vi "CAN task spawn.vi"(4 "error in (no error)":errorcluster, 7 "CANopen in":refnum<class "CANopen.lvclass">) -> (0 "error out":errorcluster, 3 "CANopen out":refnum<class "CANopen.lvclass">)   [LabVIEW 2024, in "canopen.lvlib" / "CANopen.lvclass"]
doc: "Spawns the \"CAN task\" VI with the provided arguments."
uses:
  CANopen.lvclass
  CANopen.lvclass/CANopen.ctl
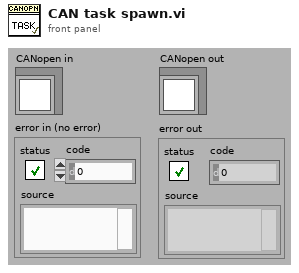
[diagram p1: front panel]
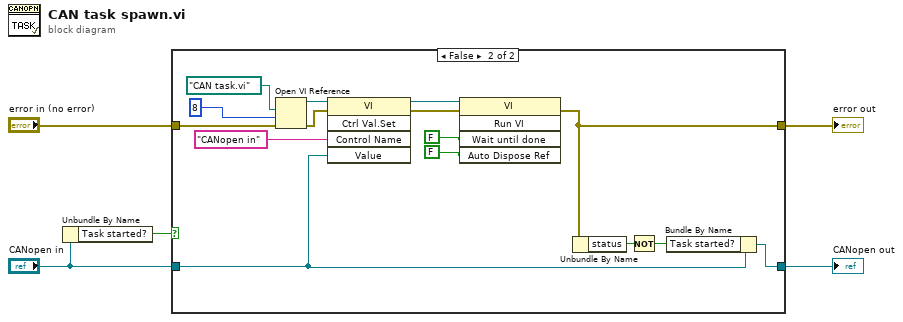
[diagram p0: block diagram]
diagram:
  n1 = Unbundle By Name("CANopen in") -> ("Task started?"=w1:bool)
  n2 = case shown="False" w1 {
    tunnel: "error in (no error)" -> [w7 w13]
    tunnel: "CANopen in" -> [w6 w12]
    tunnel: [w7 w11] -> w4
    tunnel: [w6 w8] -> w3
    frame True {
    }
    frame False {
      n3 = Open VI Reference(vi path=path "CAN task.vi", options=8, error in (no error)=w13) -> (vi reference=w18:refnum<vi>, error out=w19:errorcluster)  [unwired: 3 out]
      n4 = invoke class="VI" method="Ctrl Val.Set"(reference=w18, error in=w19, "Control Name"="CANopen in", "Value"=w12) -> (reference out=w20:refnum<vi>, error out=w21:errorcluster)  [unwired: 1 in, 3 out]
      n5 = invoke class="VI" method="Run VI"(reference=w20, error in=w21, "Wait until done"=FALSE ("Wait Until Done"), "Auto Dispose Ref"=FALSE ("Auto Dispose Reference")) -> (error out=w11:errorcluster)  [unwired: 1 in, 4 out]
      n6 = Unbundle By Name(w11) -> ("status"=w10:bool)
      n7 = Not(x=w10) -> (.not. x?=w9:bool)
      n8 = Bundle By Name(cluster=w12, "Task started?"=w9) -> (w8:refnum<class "CANopen.lvclass">)
    }
  }
  "error out" <- w4
  "CANopen out" <- w3
